vi "數位濾波版.vi"() -> ()   [LabVIEW 2010]
uses:
  <vilib>/Analysis/3filter.llb/Filter Passband Type.ctl
  <vilib>/DAQmx/read.llb/DAQmx Read (Analog DBL 1Chan 1Samp).vi
  <vilib>/DAQmx/write.llb/DAQmx Write (Analog DBL 1Chan 1Samp).vi
  <vilib>/DAQmx/create/channels.llb/DAQmx Create Channel (AI-Voltage-Basic).vi
  <vilib>/DAQmx/configure/timing.llb/DAQmx Timing (Sample Clock).vi
  <vilib>/DAQmx/create/channels.llb/DAQmx Create Channel (AO-Voltage-Basic).vi
  <vilib>/daqmx/miscellaneous.llb/DAQmx Fill In Error Info.vi
  <vilib>/Analysis/3filter.llb/Butterworth Filter (DBL).vi
  <vilib>/Analysis/NI_AALBase.lvlib
panel:
  in  "濾波?":bool
  in  "low cutoff freq: fl":dbl=200.0 format="%0.4f"
  out "理想迴圈時間":dbl
  out "延遲警告":bool
  in  "濾波階數":i32=1
  out "Waveform Graph":dbl[][](graph)
  out "當下DC值":dbl
  in  "DAQ input":tag
  in  "DAQ output":tag
  in  "平均數":i32=1
  in  "ÂoDC«á©ñ¤j":dbl=1.0
  in  "Kp":dbl=150.0
  out "當下誤差":dbl=0.1 format="%#_13g"
  out "模擬輸入x(t)":dbl[][](graph)
  out "理想與FIR輸出":dbl[][](graph)
  out "message":string=" INSTRUCTIONS:\r\rNormal Use:  When using subVIs that incorporate the error in/error out (or error I/O) structure, place this handler where you want to inform the user of an error, typically at the end of the I/O data path, as the last action of the program.  If the error in error? is ERROR, the handler creates a message describing the error and its source.  If the type of dialog = 1 (default), the message is displayed to the user, who can only acknowedge it.  If the type = 2, the user can acknowledge the message or abort execution; aborting a program with active I/O is not recommended.  If the type = 0, no message is displayed; this is used to process the error programmatically, and the error out cluster elements are wired to individual terminals for that reason.  \r\rOther Use:\n\r\nlocal testing.  To test the error code of a subVI or function that does not have the error I/O structure, you can wire its error code and a source string to the local error code and error source inputs.  If error in error? indicates no error and error code is not equal to 0, the local code and source are substituted for the error in values, and error? is set TRUE (ERROR)."
  out "誤差":dbl(graph)
  out "while平均運行時間":dbl
  in  "取樣頻率":dbl=9000.0 min=1.0 max=20000.0 step=1.0
  in  "stop":bool
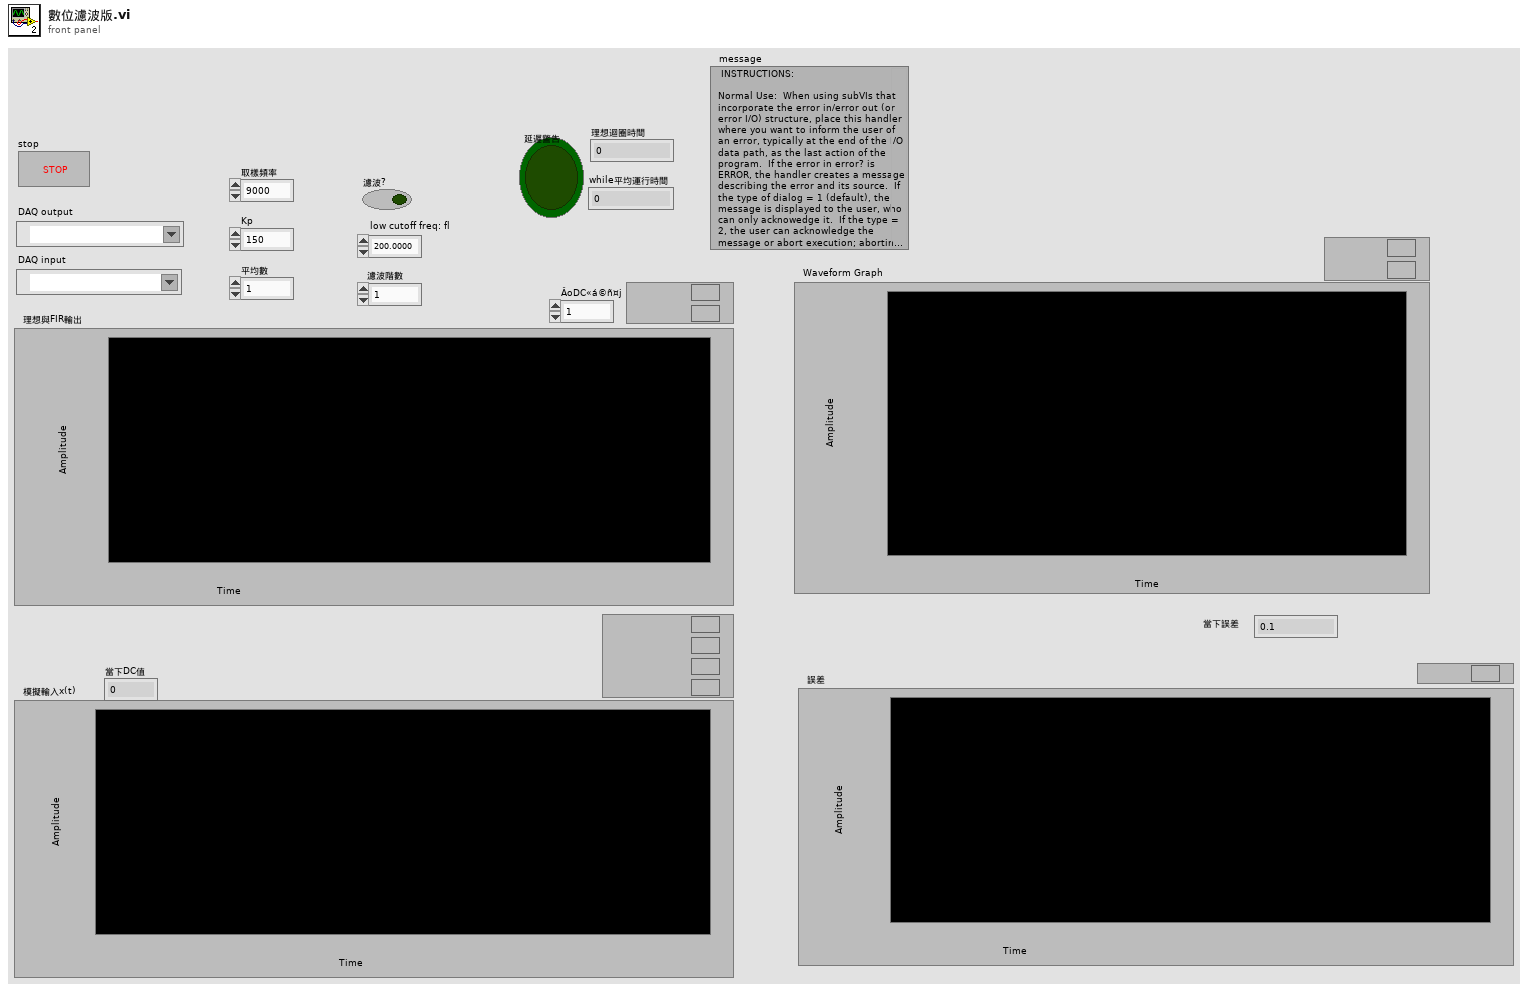
[diagram p1: front panel]
types:
  T1 = typedef "NI_AALBase.lvlib/Filter Passband Type.ctl" = enum32{"Lowpass", "Highpass", "Bandpass", "Bandstop"}
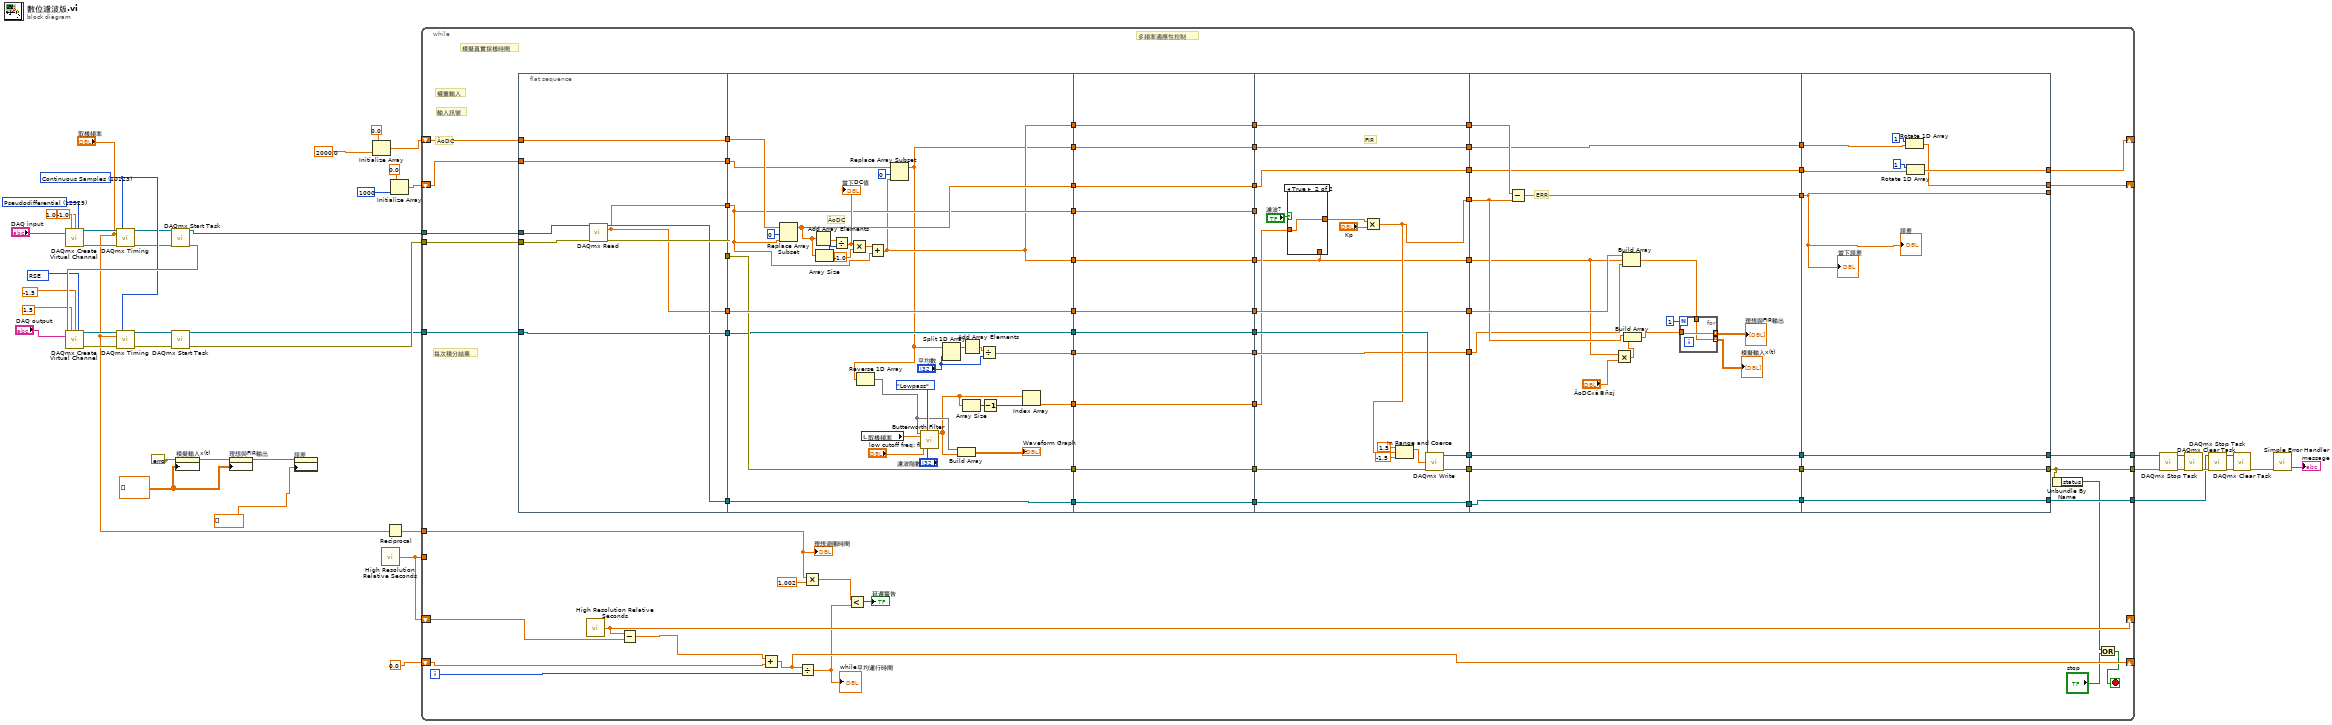
[diagram p0: block diagram]
diagram:
  w34 = 10123 items=["Finite Samples"=10178, "Continuous Samples"=10123, "Hardware Timed Single Point"=12522] ("sample mode")
  w31 = 10083 items=["Default"=-1, "RSE"=10083, "Differential"=10106, "Pseudodifferential"=12529] ("output terminal configuration")
  w30 = 12529 items=["default"=-1, "RSE"=10083, "NRSE"=10078, "Differential"=10106, "Pseudodifferential"=12529] ("input terminal configuration")
  w38 = dbl[][] [] ("History Data")
  n1 = call-poly <vilib>:"DAQmx Create Virtual Channel.vi"("maximum value"=1.0, "minimum value"=-1.0, "input terminal configuration"=w30, "physical channels"="DAQ input") -> ("task out"=w22:refnum<k21>, "error out"=w25:errorcluster)  [unwired: 10 in]
  n2 = call-poly <vilib>:"DAQmx Timing.vi"("task/channels in"=w22, "sample mode"=w34, "rate"="取樣頻率", "error in"=w25) -> ("task out"=w23:refnum<k21>, "error out"=w24:errorcluster)  [unwired: 10 in]
  n3 = call <vilib>:"DAQmx Start Task.vi"("task/channels in"=w23, "error in"=w24) -> ("task out"=w21:refnum<k21>, "error out"=w37:errorcluster)  [unwired: 12 in]
  n4 = call-poly <vilib>:"DAQmx Create Virtual Channel.vi"("maximum value"=1.5, "minimum value"=-1.5, "output terminal configuration"=w31, "physical channels"="DAQ output", "error in"=w37) -> ("task out"=w29:refnum<k21>, "error out"=w26:errorcluster)  [unwired: 9 in]
  n5 = call-poly <vilib>:"DAQmx Timing.vi"("task/channels in"=w29, "sample mode"=w34, "rate"="取樣頻率", "error in"=w26) -> ("task out"=w28:refnum<k21>, "error out"=w27:errorcluster)  [unwired: 10 in]
  n6 = call <vilib>:"DAQmx Start Task.vi"("task/channels in"=w28, "error in"=w27) -> ("task out"=w19:refnum<k21>, "error out"=w20:errorcluster)  [unwired: 12 in]
  n7 = property on="模擬輸入x(t)" class="WFChart (strict)"(error in=errorcluster {"status"=FALSE, "code"=0, "source"=""} ("error constant"), "History Data"=w38) -> (error out=w42:errorcluster)  [unwired: 1 in, 1 out]
  n8 = property on="理想與FIR輸出" class="WFChart (strict)"(error in=w42, "History Data"=w38) -> (error out=w43:errorcluster)  [unwired: 1 in, 1 out]
  n9 = property on="誤差" class="WFChart (strict)"(error in=w43, "History Data"=dbl[] []) -> ()  [unwired: 1 in, 2 out]
  n10 = Initialize Array(0.0 ("element"), 2000.0 ("y")) -> (w7:dbl[])
  n11 = call <vilib>:"High Resolution Relative Seconds.vi"() -> ("relative seconds"=w46:dbl)
  n12 = Reciprocal(x="取樣頻率") -> (1/x=w1:dbl)
  n13 = Initialize Array(0.0 ("element"), 1000 ("dimension size")) -> (w5:dbl[])
  n14 = while {
    tunnel: w46 -> [_]
    shift-right: [w110] -> _
    shift-left: w46 -> [w109]
    shift-right: [w111] -> _
    shift-left: 0.0 -> [w113]
    shift-right: [w101] -> _
    shift-left: w7 -> [w103]
    tunnel: w21 -> [w97]
    tunnel: w20 -> [w96]
    tunnel: w19 -> [w95]
    tunnel: [w91] -> w13
    tunnel: [w82] -> w12
    tunnel: [w85] -> w11
    shift-right: [w55] -> _
    shift-left: w5 -> [w60]
    tunnel: w1 -> [w51]
    i -> [w112]
    stop <- w84 stop-if-true
    # "每次積分結果"
    # "權重輸入"
    # "輸入訊號"
    # "ÂoDC"
    # "模擬真實採樣時間"
    # "多頻率適應性控制"
    n15 = flat-sequence {
      tunnel: [w116] -> w115
      tunnel: [w116] -> w107
      tunnel: [w120] -> w106
      tunnel: w103 -> [w123]
      tunnel: [w123] -> w102
      tunnel: w97 -> [w122]
      tunnel: w96 -> [w121]
      tunnel: w95 -> [w119]
      tunnel: [w119] -> w94
      tunnel: [w118] -> w88
      tunnel: [w117] -> w61
      tunnel: w60 -> [w117]
      tunnel: w115 -> [w136]
      tunnel: [w153] -> w79
      tunnel: [w154] -> w77
      tunnel: w107 -> [w154]
      tunnel: w106 -> [w153]
      tunnel: [w135] -> w75
      tunnel: w102 -> [w151]
      tunnel: [w140] -> w73
      tunnel: [w135] -> w71
      tunnel: [w141] -> w69
      tunnel: [w143] -> w67
      tunnel: w94 -> [w143]
      tunnel: [w142] -> w65
      tunnel: w88 -> [w142]
      tunnel: [w136] -> w63
      tunnel: w61 -> [w137]
      tunnel: [w131] -> w56
      tunnel: [w132] -> w54
      tunnel: w79 -> [w165]
      tunnel: [w165] -> w78
      tunnel: w77 -> [w164]
      tunnel: [w164] -> w76
      tunnel: w75 -> [w163]
      tunnel: [w163] -> w74
      tunnel: w73 -> [w162]
      tunnel: [w162] -> w72
      tunnel: w71 -> [w161]
      tunnel: [w161] -> w70
      tunnel: w69 -> [w160]
      tunnel: [w160] -> w68
      tunnel: w67 -> [w159]
      tunnel: [w159] -> w66
      tunnel: w65 -> [w158]
      tunnel: [w158] -> w64
      tunnel: w63 -> [w157]
      tunnel: [w157] -> w62
      tunnel: [w156] -> w57
      tunnel: w56 -> [w156]
      tunnel: w54 -> [w155]
      tunnel: [w155] -> w53
      tunnel: w78 -> [w180]
      tunnel: [w170] -> w108
      tunnel: w76 -> [w170]
      tunnel: [w183] -> w105
      tunnel: w74 -> [w183]
      tunnel: [w172] -> w104
      tunnel: [w182] -> w99
      tunnel: w72 -> [w182]
      tunnel: w70 -> [w166]
      tunnel: [w166] -> w98
      tunnel: w68 -> [w171]
      tunnel: w66 -> [w181]
      tunnel: [w179] -> w92
      tunnel: [w178] -> w90
      tunnel: w64 -> [w177]
      tunnel: [w177] -> w87
      tunnel: [w171] -> w80
      tunnel: w62 -> [_]
      tunnel: [w173] -> w58
      tunnel: w57 -> [w173]
      tunnel: w53 -> [w168]
      tunnel: [w201] -> w114
      tunnel: w108 -> [w199]
      tunnel: w105 -> [w200]
      tunnel: w104 -> [w197]
      tunnel: [w189] -> w100
      tunnel: w99 -> [w189]
      tunnel: w98 -> [w196]
      tunnel: [w193] -> w93
      tunnel: w92 -> [w193]
      tunnel: w90 -> [w192]
      tunnel: [w192] -> w89
      tunnel: w87 -> [w191]
      tunnel: [w191] -> w86
      tunnel: w80 -> [w190]
      tunnel: [w187] -> w59
      tunnel: w58 -> [w187]
      tunnel: w114 -> [w216]
      tunnel: [w216] -> _
      tunnel: [w214] -> w101
      tunnel: w100 -> [w213]
      tunnel: w93 -> [w212]
      tunnel: [w212] -> w91
      tunnel: [w211] -> w82
      tunnel: w89 -> [w211]
      tunnel: w86 -> [w210]
      tunnel: [w210] -> w85
      tunnel: w59 -> [w208]
      tunnel: [w207] -> w55
      frame #0 {
        n16 = call-poly <vilib>:"DAQmx Read.vi"("task/channels in"=w122, "error in"=w121) -> ("task out"=w118:refnum<k21>, "data"=w116:dbl, "error out"=w120:errorcluster)  [unwired: 11 in]
      }
      frame #1 {
        # "ÂoDC"
        n17 = Replace Array Subset(array=w151, new element=w136, index=0) -> (w140:dbl[])
        n18 = Add Array Elements(numeric array=w140) -> (sum=w150:dbl)
        n19 = Array Size(array=w140) -> (size(s)=w149:i32)
        n20 = Divide(x=w150, y=w149) -> (x/y=w148:dbl)
        "當下DC值" <- w148
        n21 = Multiply(x=w148, y=-1.0) -> (x*y=w146:dbl)
        n22 = local read "取樣頻率"() -> (w134:dbl)
        n23 = Add(x=w146, y=w136) -> (x+y=w135:dbl)
        n24 = Replace Array Subset(array=w137, new element=w135, index=0) -> (w131:dbl[])
        n25 = Reverse 1D Array(array=w131) -> (reversed array=w130:dbl[])
        n26 = call-poly <vilib>:"Butterworth Filter.vi"("order"="濾波階數", "filter type"=Filter_Passband_Type."Lowpass", "low cutoff freq: fl"="low cutoff freq: fl", "sampling freq: fs"=w134, "X"=w130) -> ("Filtered X"=w129:dbl[])  [unwired: 3 in, 1 out]
        n27 = Split 1D Array(array=w131, index="平均數") -> (first subarray=w139:dbl[])  [unwired: 1 out]
        n28 = Build Array(w130, w129) -> (→"Waveform Graph":dbl[][])
        n29 = Array Size(array=w129) -> (size(s)=w128:i32)
        n30 = Add Array Elements(numeric array=w139) -> (sum=w145:dbl)
        n31 = Divide(x=w145, y="平均數") -> (x/y=w141:dbl)
        n32 = Decrement(x=w128) -> (x-1=w127:i32)
        n33 = Index Array(array=w129, index=w127) -> (element=w132:dbl)
      }
      frame #2 {
      }
      frame #3 {
        # "FIR"
        n34 = case shown="True" "濾波?" {
          tunnel: w168 -> [_ w186]
          tunnel: [w185 w186] -> w167
          tunnel: w166 -> [w185 _]
          frame False {
          }
          frame True {
          }
        }
        n35 = Multiply(x=w167, y="Kp") -> (x*y=w172:dbl)
        n36 = In Range and Coerce(upper limit=1.5, x=w172, lower limit=-1.5) -> (coerced(x)=w176:dbl)  [unwired: 1 out]
        n37 = call-poly <vilib>:"DAQmx Write.vi"("task/channels in"=w181, "data"=w176, "error in"=w180) -> ("task out"=w179:refnum<k21>, "error out"=w178:errorcluster)  [unwired: 10 in, 1 out]
      }
      frame #4 {
        # "ERR"
        n38 = Subtract(x=w200, y=w197) -> (x-y=w201:dbl)
        n39 = Multiply(x=w196, y="ÂoDC«á©ñ¤j") -> (x*y=w194:dbl)
        n40 = Build Array(w199, w196, w190) -> (w198:dbl[])
        n41 = Build Array(w197, w194) -> (w188:dbl[])
        n42 = for {
          N: 1 -> [_]
          tunnel: [w206] -> w202 mode=indexing
          tunnel: w188 -> [w206]
          tunnel: [w205] -> w203 mode=indexing
          tunnel: w198 -> [w205]
        }
        "理想與FIR輸出" <- w202
        "模擬輸入x(t)" <- w203
      }
      frame #5 {
        n43 = Rotate 1D Array(1:w208, 2:1 ("n")) -> (0:w207:dbl[])
        n44 = Rotate 1D Array(1:w213, 2:1 ("n")) -> (0:w214:dbl[])
        "誤差" <- w216
        "當下誤差" <- w216
      }
    }
    n45 = call <vilib>:"High Resolution Relative Seconds.vi"() -> ("relative seconds"=w110:dbl)
    n46 = Subtract(x=w110, y=w109) -> (x-y=w52:dbl)
    n47 = Add(x=w52, y=w113) -> (x+y=w111:dbl)
    n48 = Divide(x=w111, y=w112) -> (x/y=w48:dbl)
    "while平均運行時間" <- w48
    n49 = Multiply(x=w51, y=1.002) -> (x*y=w49:dbl)
    n50 = Less?(x=w49, y=w48) -> (x < y?=→"延遲警告":bool)
    n51 = Unbundle By Name(w82) -> ("status"=w81:bool)
    n52 = Or(x=w81, y="stop") -> (x .or. y?=w84:bool)
    "理想迴圈時間" <- w51
  }
  n53 = call <vilib>:"DAQmx Stop Task.vi"("task/channels in"=w13, "error in"=w12) -> ("task out"=w14:refnum<k21>, "error out"=w15:errorcluster)  [unwired: 12 in]
  n54 = call <vilib>:"DAQmx Clear Task.vi"("task in"=w14, "error in"=w15) -> ("error out"=w18:errorcluster)  [unwired: 13 in]
  n55 = call <vilib>:"DAQmx Stop Task.vi"("task/channels in"=w11, "error in"=w18) -> ("task out"=w17:refnum<k21>, "error out"=w16:errorcluster)  [unwired: 12 in]
  n56 = call <vilib>:"DAQmx Clear Task.vi"("task in"=w17, "error in"=w16) -> ("error out"=w10:errorcluster)  [unwired: 13 in]
  n57 = call <vilib>:"Simple Error Handler.vi"("error in (no error)"=w10) -> ("message"=→"message":string)  [unwired: 4 in, 4 out]
